vi "IDS_displacement_getAbsolutePositions.vi"(0 "deviceHandle":i32, 11 "error in (no error)":errorcluster) -> (4 "deviceHandle out":i32, 6 "position axis 1":i64, 8 "position axis 2":i64, 10 "position axis 3":i64, 15 "error out":errorcluster)   [LabVIEW 2016]
doc: "int IDS_DLL IDS_displacement_getAbsolutePositions(int64_t *position0, int64_t * position1, int64_t * position2);"
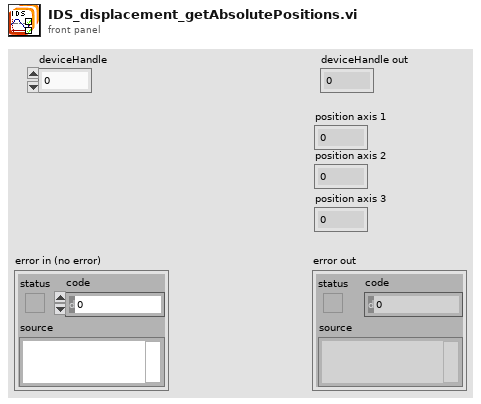
[diagram p1: front panel]
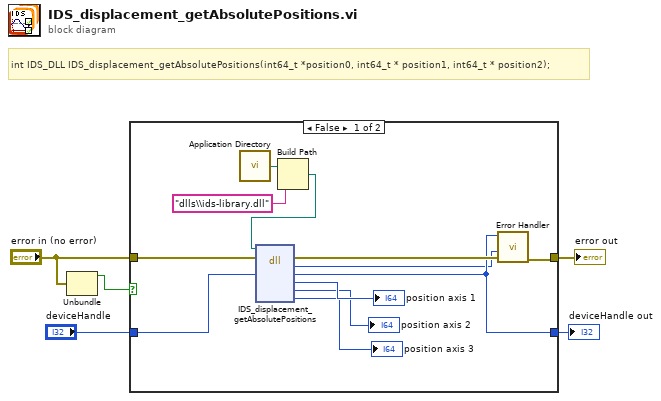
[diagram p0: block diagram]
diagram:
  # "int IDS_DLL IDS_displacement_getAbsolutePositions(int64_t *position0, int64_t * position1, int64_t * position2);"
  n1 = Unbundle("error in (no error)") -> ("status"=w1:bool)  [unwired: 2 out]
  n2 = case shown="False" w1 {
    tunnel: "error in (no error)" -> [w17 w19]
    tunnel: [w12 w19] -> w5
    tunnel: "deviceHandle" -> [w11 w18]
    tunnel: [w10 w18] -> w3
    frame False {
      n3 = call <vilib>:"Application Directory.vi"() -> ("Application Directory"=w8:path)
      n4 = Build Path(base path=w8, name or relative path="dlls\\ids-library.dll" ("ipAddress")) -> (appended path=w6:path)
      n5 = dll-call lib="C:/Users/matheus/Desktop/LabVIEW_Draft_V1.6.0/dlls/ids-library.*" fn="IDS_displacement_getAbsolutePositions"(path in=w6, error in=w17, "deviceHandle"=w11) -> (error out=w13:errorcluster, "Error Code"=w9:i32, "deviceHandle"=w10:i32, "Position Axis 1"=→"position axis 1":i64, "Position Axis 2"=→"position axis 2":i64, "Position Axis 3"=→"position axis 3":i64)  [unwired: 4 in, 1 out]
      n6 = call "Error Handler.vi"("error in (no error)"=w13, "error code"=w9, "deviceHandle"=w10) -> ("error out"=w12:errorcluster)  [unwired: 7 in, 1 out]
    }
    frame True {
    }
  }
  "error out" <- w5
  "deviceHandle out" <- w3
